vi "GetRaster.vi"(0 "Scan in":refnum<class "Scan.lvclass">, 1 "Camera in":refnum<class "Camera.lvclass">, 2 "Galvo Array":refnum<class "Galvonometer.lvclass">[](array[class]), 3 "error in (no error)":errorcluster) -> (4 "Return A":dbl, 5 "cropLinesOut":dbl, 6 "Delay A":dbl, 7 "Galvo Array":dbl[][](array[numeric]), 8 "error IO":errorcluster)   [LabVIEW 2017]
uses:
  classes/Scans/Scan.lvclass
  classes/HardwareObjects/Galvonometer/Galvonometer.lvclass
  classes/HardwareObjects/Camera/Camera.lvclass
  classes/Scans/Scan.lvclass/Scan.ctl
  classes/HardwareObjects/Galvonometer/Galvonometer.lvclass/Galvonometer.ctl
  classes/Scans/Read A scans.vi
  classes/Scans/Read B scans.vi
  classes/Scans/Read Bidirectional.vi
  classes/Scans/Read C scans.vi
  classes/Scans/Read Repeat B scans.vi
  classes/Scans/Read Scan Angle (degrees).vi
  classes/Scans/Read Scan Pattern.vi
  classes/Scans/Read X FOV (degrees).vi
  classes/Scans/Read X offset (degrees).vi
  classes/Scans/Read Y FOV (degrees).vi
  classes/Scans/Read Y offset (degrees).vi
  <vilib>/Analysis/1siggen.llb/Ramp Pattern by Samples.vi
  classes/HardwareObjects/Galvonometer/Read Output Scale Factor (V_degrees).vi
  classes/Scans/Read Total A-scans per volume.vi
  classes/Scans/Read Total B-Scans.vi
  <vilib>/Utility/file.llb/Write Delimited Spreadsheet (DBL).vi
  <vilib>/Analysis/NI_AALBase.lvlib
panel:
  in  "Crop Lines":dbl=1.0 format="%#_13g"
  out "getRasterProfile":dbl
  in  "Read scan parameters":bool
  in  "Display Raster":bool
  out "Y offset (degrees)":dbl
  out "Y FOV (degrees)":dbl
  out "X offset (degrees)":dbl
  out "X FOV (degrees)":dbl
  out "Scan Pattern":string
  out "Scan Angle (degrees)":dbl
  out "Repeat B scans":dbl
  out "C scans":dbl
  out "Bidirectional":bool
  out "B scans":dbl
  out "A scans":dbl
  out "Raster":dbl[][](graph)
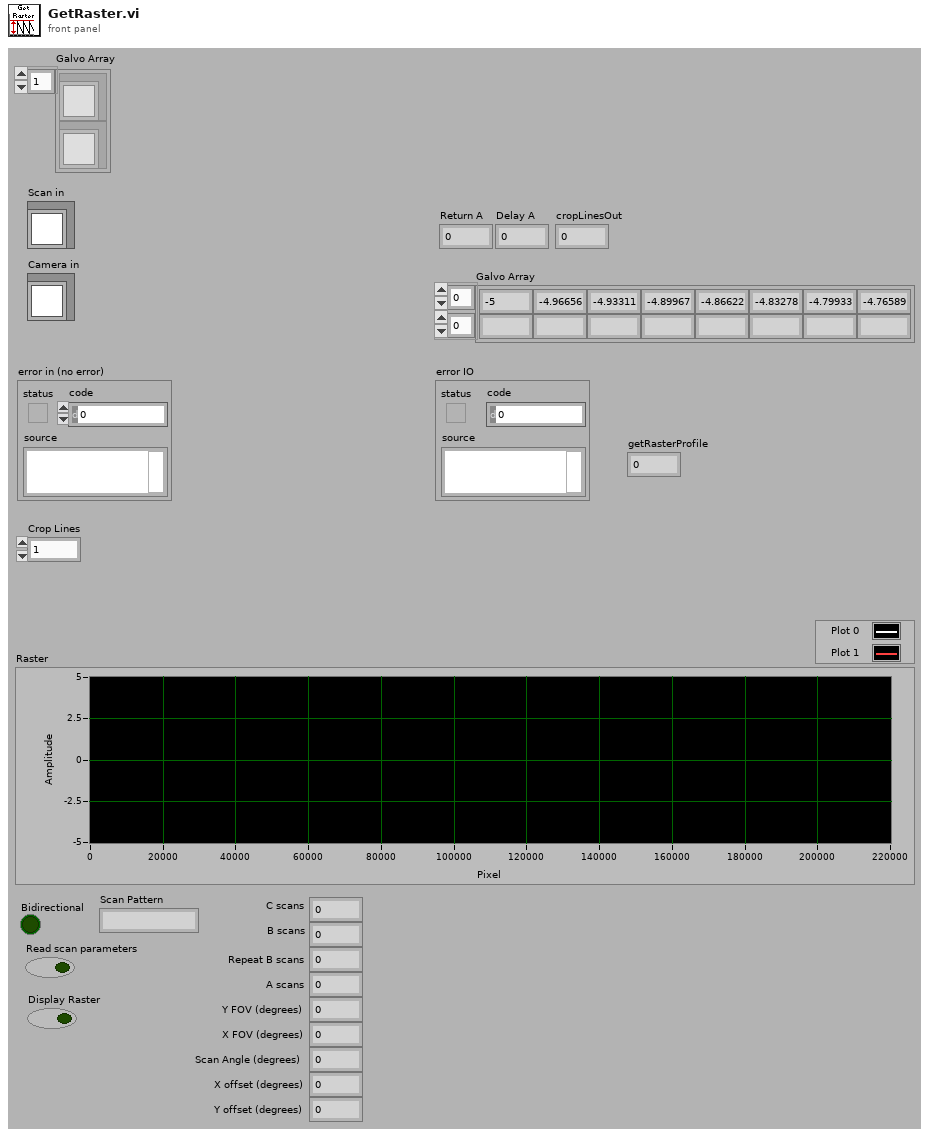
[diagram p1: front panel]
types:
  T1 = cluster{"X FOV (degrees)":dbl, "X offset (degrees)":dbl, "Y FOV (degrees)":dbl, "Y offset (degrees)":dbl}
  T2 = cluster{"X FOV (degrees)":dbl, "Y FOV (degrees)":dbl}
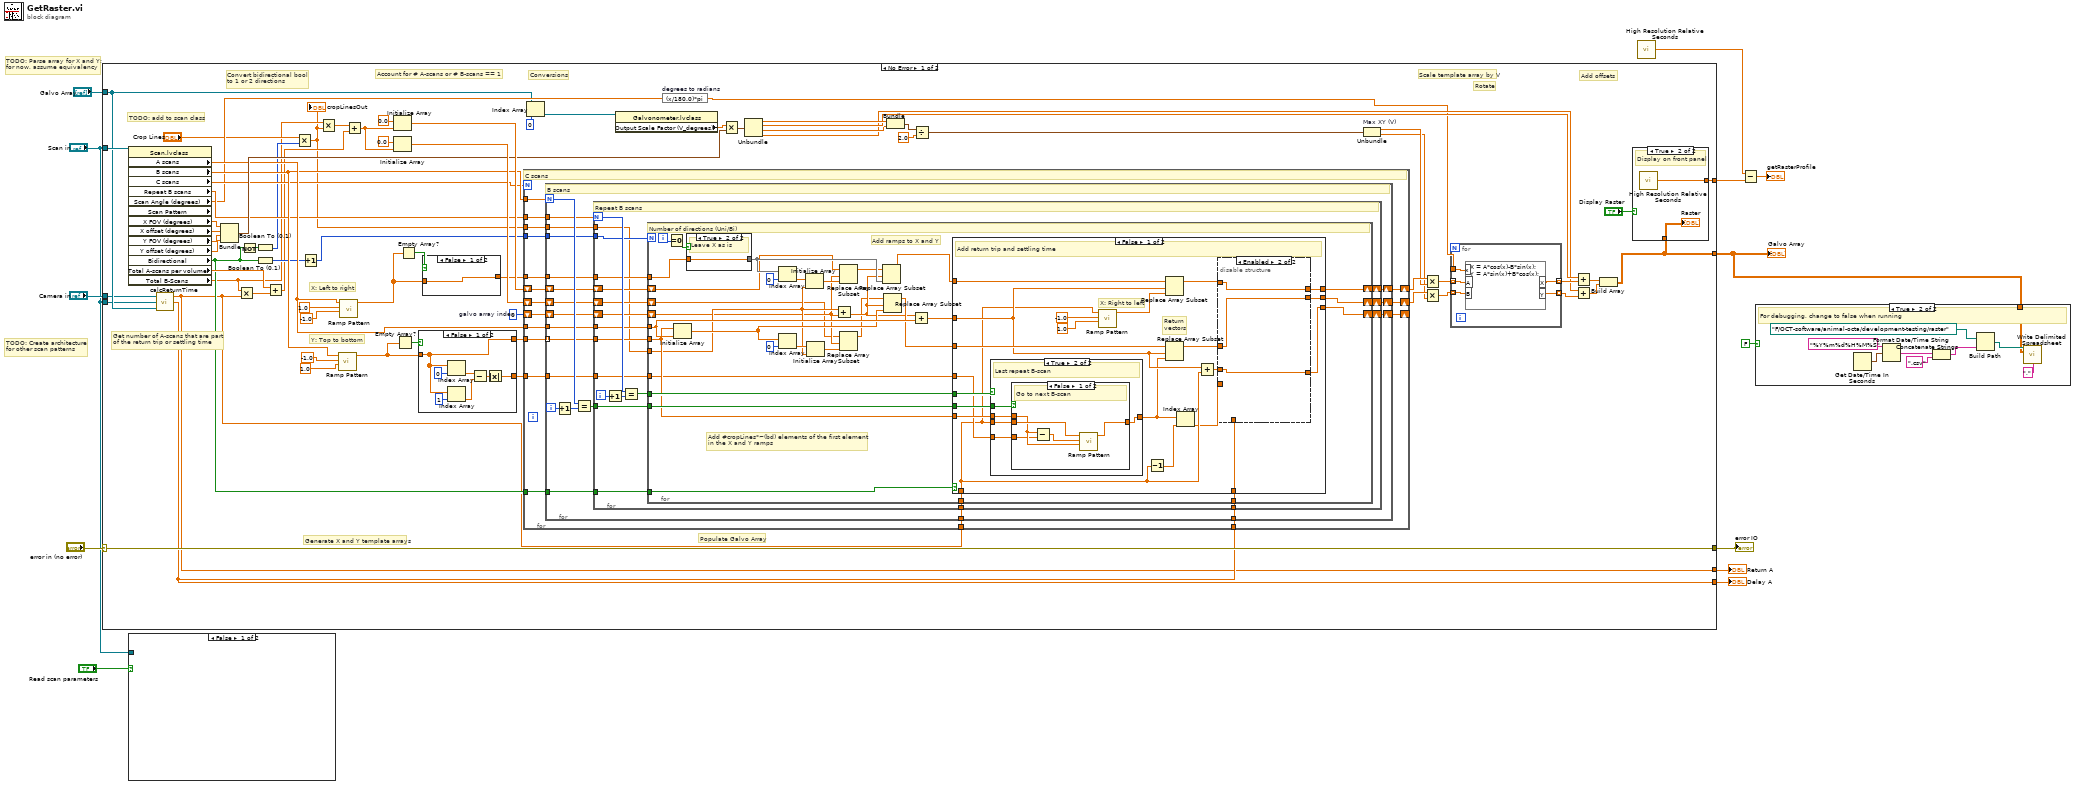
[diagram p0: block diagram]
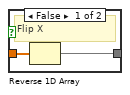
[diagram p2: hidden frame]
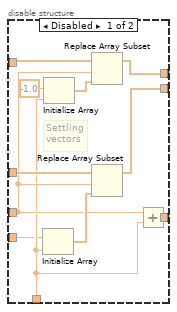
[diagram p3: hidden frame]
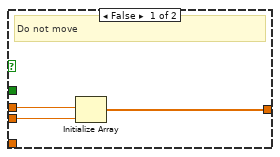
[diagram p4: hidden frame]
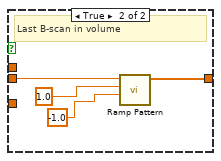
[diagram p5: hidden frame]
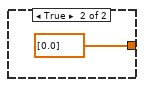
[diagram p7: hidden frame]
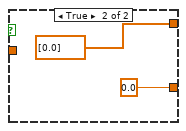
[diagram p8: hidden frame]
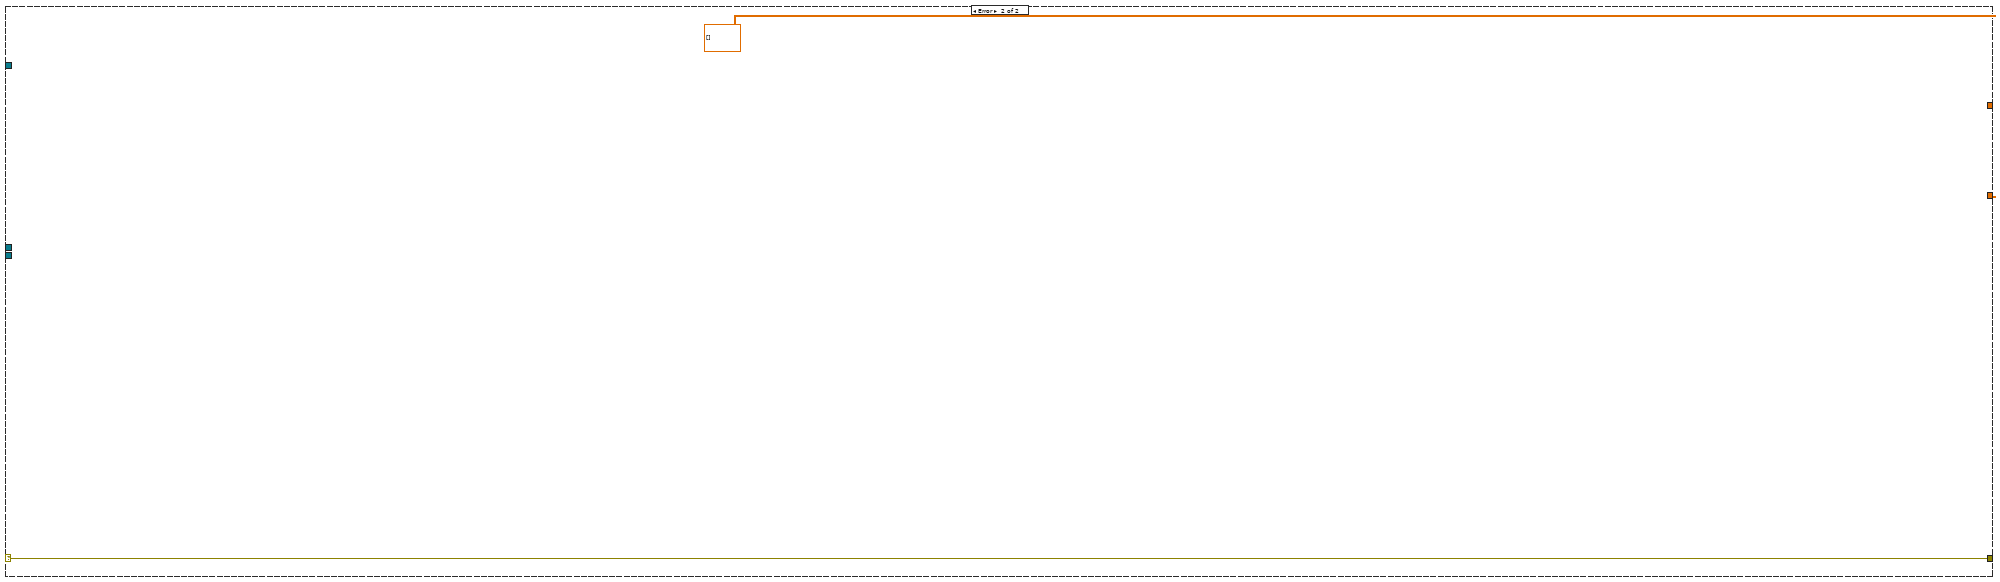
[diagram p10: hidden frame]
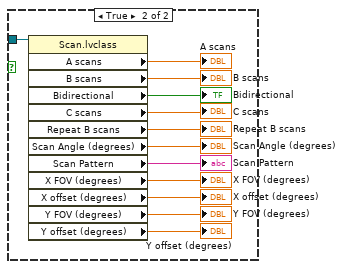
[diagram p11: hidden frame]
diagram:
  # "TODO: Create architecture\nfor other scan patterns"
  # "TODO: Parse array for X and Y;\nfor now, assume equivalency"
  n1 = case shown="No Error" "error in (no error)" {
    selector: "error in (no error)" -> [w84 w251]
    tunnel: [w84 w251] -> w13
    tunnel: [w38 dbl[][] []] -> w9
    tunnel: "Scan in" -> [w53 _]
    tunnel: "Galvo Array" -> [w36 _]
    tunnel: "Camera in" -> [w35 _]
    tunnel: "Scan in" -> [w34 _]
    tunnel: [w15 _] -> w5
    tunnel: [w26 _] -> w4
    tunnel: [w25 _] -> w2
    frame No Error {
      w77 = 0  # galvo array index
      # "TODO: add to scan class"
      # "Get number of A-scans that are part\nof the return trip or settling time"
      # "Account for # A-scans or # B-scans == 1"
      # "Convert bidirectional bool\nto 1 or 2 directions"
      # "Conversions"
      # "Add offsets"
      # "Rotate"
      # "Scale template array by V"
      # "Populate Galvo Array"
      # "Y: Top to bottom"
      # "X: Left to right"
      # "Generate X and Y template arrays"
      n2 = property class="Scan.lvclass" props=["A scans", "B scans", "C scans", "Repeat B scans", "Scan Angle (degrees)", "Scan Pattern", "X FOV (degrees)", "X offset (degrees)", "Y FOV (degrees)", "Y offset (degrees)", "Bidirectional", "Total A-scans per volume", "Total B-Scans"](reference=w53) -> ("A scans"=w50:dbl, "B scans"=w49:dbl, "C scans"=w48:dbl, "Repeat B scans"=w47:dbl, "Scan Angle (degrees)"=w46:dbl, "X FOV (degrees)"=w54:dbl, "X offset (degrees)"=w55:dbl, "Y FOV (degrees)"=w56:dbl, "Y offset (degrees)"=w57:dbl, "Bidirectional"=w22:bool, "Total A-scans per volume"=w33:dbl, "Total B-Scans"=w19:dbl)  [unwired: 1 in, 3 out]
      n3 = call "calcReturnTime.vi"("Galvo obj array"=w36, "Scan in"=w34, "Camera in"=w35) -> ("Delay A"=w26:dbl, "Inactive A"=w15:dbl)  [unwired: 1 in]
      n4 = Bundle("X FOV (degrees)"=w54, "X offset (degrees)"=w55, "Y FOV (degrees)"=w56, "Y offset (degrees)"=w57) -> (w51:T1)  [unwired: 1 in]
      n5 = Multiply(x=w19, y=w15) -> (x*y=w32:dbl)
      n6 = Not(x=w22) -> (.not. x?=w21:bool)
      n7 = Boolean To (0,1)(Boolean=w21) -> (0, 1=w20:i16)
      n8 = Boolean To (0,1)(Boolean=w22) -> (0, 1=w23:i16)
      n9 = Add(x=w33, y=w32) -> (x+y=w17:dbl)
      n10 = Multiply(x="Crop Lines", y=w20) -> (x*y=w14:dbl)
      "cropLinesOut" <- w14
      n11 = Increment(x=w23) -> (x+1=w52:i16)
      n12 = Multiply(x=w19, y=w14) -> (x*y=w18:dbl)
      n13 = call-poly <vilib>:"Ramp Pattern.vi"("start"=1.0, "end"=-1.0, "samples"=w49) -> ("Ramp Pattern"=w29:dbl[])  [unwired: 7 in, 1 out]
      n14 = call-poly <vilib>:"Ramp Pattern.vi"("start"=-1.0, "end"=1.0, "samples"=w50) -> ("Ramp Pattern"=w31:dbl[])  [unwired: 7 in, 1 out]
      n15 = Add(x=w18, y=w17) -> (x+y=w16:dbl)
      n16 = Initialize Array(0.0 ("element"), w16) -> (w75:dbl[])
      n17 = Initialize Array(0.0 ("element"), w16) -> (w78:dbl[])
      n18 = Empty Array?(array=w29) -> (empty?=w28:bool)
      n19 = Empty Array?(array=w31) -> (empty?=w30:bool)
      n20 = case shown="False" w28 {
        tunnel: w29 -> [w238 _]
        tunnel: [w238 dbl[] [0.0] ("Ramp Pattern")] -> w40
        tunnel: [w234 0.0] -> w27
        frame False {
          n21 = Index Array(array=w238, index=0) -> (element=w237:dbl)
          n22 = Index Array(array=w238, index=1) -> (element=w236:dbl)
          n23 = Subtract(x=w237, y=w236) -> (x-y=w235:dbl)
          n24 = Absolute Value(x=w235) -> (abs(x)=w234:dbl)
        }
        frame True {
        }
      }
      n25 = case shown="False" w30 {
        tunnel: w31 -> [w232 _]
        tunnel: [w232 dbl[] [0.0] ("Ramp Pattern")] -> w39
        frame False {
        }
        frame True {
        }
      }
      n26 = for {
        N: w48 -> [_]
        tunnel: w49 -> [w101]
        tunnel: w47 -> [w100]
        tunnel: w52 -> [w99]
        tunnel: w39 -> [w97]
        tunnel: w50 -> [w95]
        shift-right: [w91] -> _
        shift-left: w77 -> [w96]
        shift-right: [w94] -> w74
        shift-left: w78 -> [w98]
        shift-right: [w92] -> w73
        shift-left: w75 -> [w93]
        tunnel: w40 -> [w90]
        tunnel: w22 -> [w89]
        tunnel: w15 -> [w88]
        tunnel: w27 -> [w87]
        tunnel: w26 -> [w86]
        tunnel: w14 -> [w85]
        # "C scans"
        n27 = for {
          N: w101 -> [w121]
          tunnel: w100 -> [w120]
          tunnel: w99 -> [w119]
          tunnel: w97 -> [w118]
          tunnel: w95 -> [w116]
          shift-right: [w112] -> w91
          shift-left: w96 -> [w117]
          shift-right: [w115] -> w94
          shift-left: w98 -> [w110]
          shift-right: [w113] -> w92
          shift-left: w93 -> [w114]
          tunnel: w90 -> [w111] mode=indexing
          tunnel: w89 -> [w109]
          tunnel: w88 -> [w108]
          tunnel: w87 -> [w104]
          tunnel: w86 -> [w103]
          tunnel: w85 -> [w102]
          i -> [w107]
          # "B scans"
          n28 = Increment(x=w107) -> (x+1=w106:i32)
          n29 = Equal?(x=w121, y=w106) -> (x = y?=w105:bool)
          n30 = for {
            N: w120 -> [w141]
            tunnel: w119 -> [w140]
            tunnel: w118 -> [w139]
            tunnel: w116 -> [w137]
            shift-right: [w133] -> w112
            shift-left: w117 -> [w138]
            shift-right: [w136] -> w115
            shift-left: w110 -> [w131]
            shift-right: [w134] -> w113
            shift-left: w114 -> [w135]
            tunnel: w111 -> [w132]
            tunnel: w109 -> [w130]
            tunnel: w108 -> [w129]
            tunnel: w105 -> [w126]
            tunnel: w104 -> [w124]
            tunnel: w103 -> [w123]
            tunnel: w102 -> [w122]
            i -> [w128]
            # "Repeat B scans"
            n31 = Increment(x=w128) -> (x+1=w127:i32)
            n32 = Equal?(x=w141, y=w127) -> (x = y?=w125:bool)
            n33 = for {
              N: w140 -> [_]
              tunnel: w139 -> [w171]
              shift-right: [w167] -> w136
              shift-left: w131 -> [w150]
              tunnel: w137 -> [w170]
              shift-right: [w163] -> w133
              shift-left: w138 -> [w143]
              shift-right: [w165] -> w134
              shift-left: w135 -> [w142]
              tunnel: w132 -> [w159]
              tunnel: w130 -> [w169]
              tunnel: w129 -> [w162]
              tunnel: w126 -> [w160]
              tunnel: w125 -> [w161]
              tunnel: w124 -> [w158]
              tunnel: w123 -> [w157]
              tunnel: w122 -> [w146]
              i -> [w173]
              # "Add #cropLines*~(bd) elements of the first element\nin the X and Y ramps"
              # "Add ramps to X and Y"
              # "Number of directions (Uni/Bi)"
              n34 = Equal To 0?(x=w173) -> (x = 0?=w172:bool)
              n35 = Initialize Array(w159, w170) -> (w153:dbl[])
              n36 = case shown="True" w172 {
                tunnel: w171 -> [w175 w176]
                tunnel: [w174 w176] -> w156
                frame False {
                  # "Flip X"
                  n37 = Reverse 1D Array(array=w175) -> (reversed array=w174:dbl[])
                }
                frame True {
                  # "Leave X as is"
                }
              }
              n38 = Index Array(array=w156, index=0) -> (element=w152:dbl)
              n39 = Index Array(array=w153, index=0) -> (element=w151:dbl)
              n40 = Initialize Array(w152, w146) -> (w149:dbl[])
              n41 = Initialize Array(w151, w146) -> (w148:dbl[])
              n42 = Add(x=w146, y=w143) -> (x+y=w147:dbl)
              n43 = Replace Array Subset(array=w142, new element=w148, index=w143) -> (w144:dbl[])
              n44 = Replace Array Subset(array=w150, new element=w149, index=w143) -> (w145:dbl[])
              n45 = Replace Array Subset(array=w145, new element=w156, index=w147) -> (w168:dbl[])
              n46 = Replace Array Subset(array=w144, new element=w153, index=w147) -> (w166:dbl[])
              n47 = Add(x=w147, y=w170) -> (x+y=w164:dbl)
              n48 = case shown="False" w169 {
                tunnel: w168 -> [w195 w231]
                tunnel: [w178 w231] -> w167
                tunnel: w166 -> [w190 w230]
                tunnel: [w177 w230] -> w165
                tunnel: w164 -> [w188 w229]
                tunnel: [w183 w229] -> w163
                tunnel: w162 -> [w181 _]
                tunnel: w161 -> [w193 _]
                tunnel: w160 -> [w192 _]
                tunnel: w159 -> [w191 _]
                tunnel: w158 -> [w189 _]
                tunnel: w157 -> [w184 _]
                frame False {
                  # "Return\nvectors"
                  # "X: Right to left"
                  # "Add return trip and settling time"
                  n49 = case shown="True" w193 {
                    tunnel: w192 -> [_ w219]
                    tunnel: w191 -> [w214 w216]
                    tunnel: w181 -> [w213 w218]
                    tunnel: [w212 w217] -> w182
                    tunnel: w189 -> [_ w215]
                    frame False {
                      # "Do not move"
                      n50 = Initialize Array(w214, w213) -> (w212:dbl[])
                    }
                    frame True {
                      # "Last repeat B-scan"
                      n51 = case shown="False" w219 {
                        tunnel: w218 -> [w224 w228]
                        tunnel: [w223 w225] -> w217
                        tunnel: w216 -> [w221 _]
                        tunnel: w215 -> [w220 _]
                        frame False {
                          # "Go to next B-scan"
                          n52 = Subtract(x=w221, y=w220) -> (x-y=w222:dbl)
                          n53 = call-poly <vilib>:"Ramp Pattern.vi"("start"=w221, "end"=w222, "samples"=w224) -> ("Ramp Pattern"=w223:dbl[])  [unwired: 7 in, 1 out]
                        }
                        frame True {
                          # "Last B-scan in volume"
                          n54 = call-poly <vilib>:"Ramp Pattern.vi"("start"=-1.0, "end"=1.0, "samples"=w228) -> ("Ramp Pattern"=w225:dbl[])  [unwired: 7 in, 1 out]
                        }
                      }
                    }
                  }
                  n55 = call-poly <vilib>:"Ramp Pattern.vi"("start"=1.0, "end"=-1.0, "samples"=w181) -> ("Ramp Pattern"=w194:dbl[])  [unwired: 7 in, 1 out]
                  n56 = Decrement(x=w181) -> (x-1=w180:dbl)
                  n57 = Replace Array Subset(array=w195, new element=w194, index=w188) -> (w187:dbl[])
                  n58 = Replace Array Subset(array=w190, new element=w182, index=w188) -> (w186:dbl[])
                  n59 = Index Array(array=w182, index=w180) -> (element=w179:dbl)
                  n60 = Add(x=w188, y=w181) -> (x+y=w185:dbl)
                  n61 = disable-structure shown="Enabled" {
                    disable-tunnel: w187 -> [w208 w209]
                    disable-tunnel: w186 -> [w207 w210]
                    disable-tunnel: w185 -> [w204 w211]
                    disable-tunnel: w184 -> [w203 _]
                    disable-tunnel: [w202 w211] -> w183
                    disable-tunnel: w179 -> [w200 _]
                    disable-tunnel: [w199 w209] -> w178
                    disable-tunnel: [w198 w210] -> w177
                    frame Disabled {
                      # "Settling\nvectors"
                      n62 = Initialize Array(w200, w203) -> (w206:dbl[])
                      n63 = Initialize Array(-1.0 ("end"), w203) -> (w205:dbl[])
                      n64 = Replace Array Subset(array=w208, new element=w205, index=w204) -> (w199:dbl[])
                      n65 = Replace Array Subset(array=w207, new element=w206, index=w204) -> (w198:dbl[])
                      n66 = Add(x=w204, y=w203) -> (x+y=w202:dbl)
                    }
                    frame Enabled {
                    }
                  }
                }
                frame True {
                }
              }
            }
          }
        }
      }
      n67 = Index Array(array=w36, index=0) -> (element=w45:refnum<class "Galvonometer.lvclass">)
      n68 = property class="Galvonometer.lvclass"(reference=w45) -> ("Output Scale Factor (V_degrees)"=w43:dbl)  [unwired: 1 in, 2 out]
      n69 = expression code="(x/180.0)*pi" "degrees to radians"(w46) -> (w37:dbl)
      n70 = Multiply(x=w43, y=w51) -> (x*y=w58:T1)
      n71 = Unbundle ("All in Volts")(w58) -> ("X FOV (degrees)"=w61:dbl, "X offset (degrees)"=w60:dbl, "Y FOV (degrees)"=w59:dbl, "Y offset (degrees)"=w41:dbl)
      n72 = Bundle("X FOV (degrees)"=w61, "Y FOV (degrees)"=w59) -> (w62:T2)  [unwired: 1 in]
      n73 = Divide(x=w62, y=2.0) -> (x/y=w64:T2)
      n74 = Unbundle "Max XY (V)"(w64) -> ("X FOV (degrees)"=w66:dbl, "Y FOV (degrees)"=w65:dbl)
      n75 = Multiply(x=w74, y=w66) -> (x*y=w72:dbl[])
      n76 = Multiply(x=w73, y=w65) -> (x*y=w71:dbl[])
      n77 = for {
        tunnel: w72 -> [w249] mode=indexing
        tunnel: w37 -> [w248]
        tunnel: [w247] -> w69 mode=indexing
        tunnel: w71 -> [w246] mode=indexing
        tunnel: [w245] -> w42 mode=indexing
        n78 = formula code="X = A*cos(x)-B*sin(x);\nY = A*sin(x)+B*cos(x);"("x"=w248, "A"=w249, "B"=w246) -> ("X"=w247:dbl, "Y"=w245:dbl)
      }
      n79 = Add(x=w60, y=w69) -> (x+y=w68:dbl[])
      n80 = Add(x=w41, y=w42) -> (x+y=w67:dbl[])
      n81 = Build Array(w68, w67) -> (w38:dbl[][])
      n82 = case shown="True" "Display Raster" {
        tunnel: w38 -> [_ w244]
        tunnel: [_ w243] -> w25
        frame False {
        }
        frame True {
          # "Display on front panel"
          n83 = call <vilib>:"High Resolution Relative Seconds.vi"() -> ("relative seconds"=w243:dbl)
          "Raster" <- w244
        }
      }
    }
    frame Error {
    }
  }
  "error IO" <- w13
  "Galvo Array" <- w9
  "Return A" <- w5
  "Delay A" <- w4
  n84 = case shown="False" "Read scan parameters" {
    tunnel: "Scan in" -> [_ w263]
    frame False {
    }
    frame True {
      n85 = property class="Scan.lvclass"(reference=w263) -> ("A scans"=→"A scans":dbl, "B scans"=→"B scans":dbl, "Bidirectional"=→"Bidirectional":bool, "C scans"=→"C scans":dbl, "Repeat B scans"=→"Repeat B scans":dbl, "Scan Angle (degrees)"=→"Scan Angle (degrees)":dbl, "Scan Pattern"=→"Scan Pattern":string, "X FOV (degrees)"=→"X FOV (degrees)":dbl, "X offset (degrees)"=→"X offset (degrees)":dbl, "Y FOV (degrees)"=→"Y FOV (degrees)":dbl, "Y offset (degrees)"=→"Y offset (degrees)":dbl)  [unwired: 1 in, 2 out]
    }
  }
  n86 = call <vilib>:"High Resolution Relative Seconds.vi"() -> ("relative seconds"=w3:dbl)
  n87 = Subtract(x=w3, y=w2) -> (x-y=→"getRasterProfile":dbl)
  n88 = case shown="True" FALSE {
    tunnel: w9 -> [_ w264]
    frame False {
    }
    frame True {
      # "For debugging, change to false when running"
      n89 = Get Date/Time In Seconds() -> (seconds since 1Jan1904=w272:timestamp)
      n90 = Format Date/Time String(time format string (%c)="%Y%m%d%H%M%S", seconds (now)=w272) -> (date/time string=w268:string)  [unwired: 1 in]
      n91 = Concatenate Strings(w268, ".csv" ("string")) -> (w267:string)
      n92 = Build Path(base path=path "F:/OCT-software/animal-octa/development-testing/raster", name or relative path=w267) -> (appended path=w265:path)
      n93 = call-poly <vilib>:"Write Delimited Spreadsheet.vi"("file path (dialog if empty)"=w265, "2D data"=w264, "delimiter (\\t)"="," ("delimiter (\\t)")) -> ()  [unwired: 11 in, 2 out]
    }
  }
